vi "Marshal.vi"(8 "error in (no error)":errorcluster, 11 "int32 in":refnum<class "string.lvclass">) -> (0 "error out":errorcluster, 2 "Buffer":u8[](array[numeric]), 3 "int32 out":refnum<class "string.lvclass">)   [LabVIEW 2020, in "Protobuf RAW.lvlib" / "string.lvclass"]
uses:
  string.lvclass
  string.lvclass/string.ctl
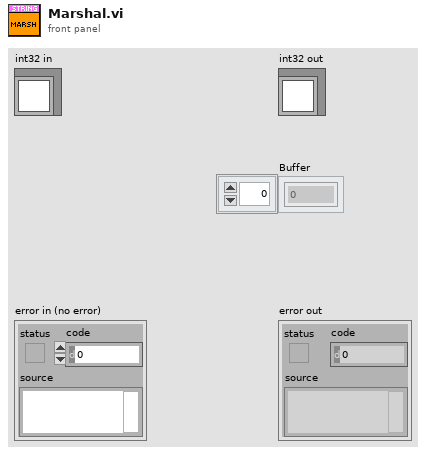
[diagram p1: front panel]
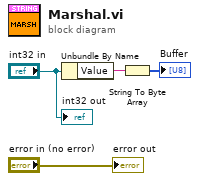
[diagram p0: block diagram]
diagram:
  n1 = Unbundle By Name("int32 in") -> ("Value"=w1:string)
  n2 = String To Byte Array(string=w1) -> (unsigned byte array=→"Buffer":u8[])
  "error out" <- "error in (no error)"
  "int32 out" <- "int32 in"
